vi "Inicializar_Control_File(SubVI).vi"(8 "error in":errorcluster, 10 "tdms file":refnum<k34>, 11 "Offsets":i64[](array[numeric])) -> (0 "error out":errorcluster)   [LabVIEW 2015]
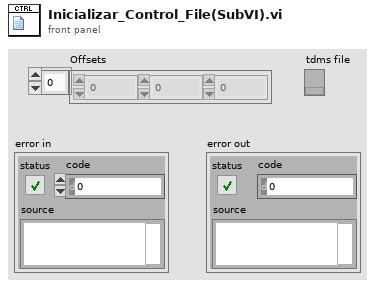
[diagram p1: front panel]
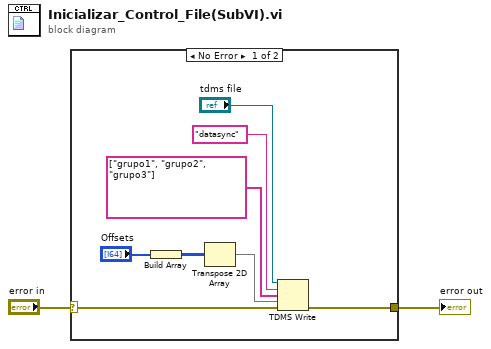
[diagram p0: block diagram]
diagram:
  n1 = case shown="No Error" "error in" {
    selector: "error in" -> [w3 w11]
    tunnel: [w5 w11] -> w2
    frame No Error {
      n2 = Build Array("Offsets") -> (w9:i64[][])
      n3 = Transpose 2D Array(2D array=w9) -> (transposed array=w10:i64[][])
      n4 = TDMS Write(0:"tdms file", 5:"datasync" ("group name in"), 7:string[] ["grupo1", "grupo2", "grupo3"], 9:w10, 11:w3) -> (15:w5:errorcluster)  [unwired: 1 in, 3 out]
    }
    frame Error {
    }
  }
  "error out" <- w2
